vi "Prober_InitialiseUI.vi"(8 "error in (no error)":errorcluster, 11 "ProbeStationControl in":refnum<class "ProbeStationControl.lvclass">) -> (0 "error out":errorcluster, 3 "ProbeStationControl out":refnum<class "ProbeStationControl.lvclass">)   [LabVIEW 2018, in "ProbeStationControl.lvclass"]
uses:
  ProbeStationControl.lvclass
  ProbeStationControl.lvclass/ProbeStationControl.ctl
panel:
  in  "Needles Clear":bool
  in  "Nucleus":bool
  in  "Stop Button":bool
  out "Ref No.":u32
  # "Starting Probe Station Control Interface"
  # "Before continuing, please confirm the following:"
  # "1. NUCLEUS is activiated"
  # "2. No device on chuck and needles are clear"
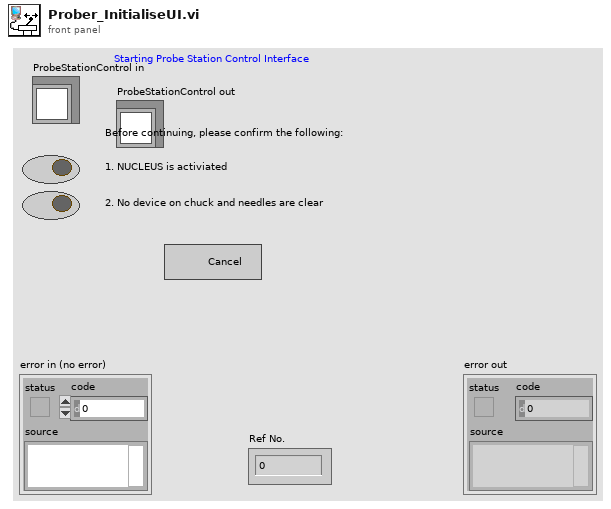
[diagram p1: front panel]
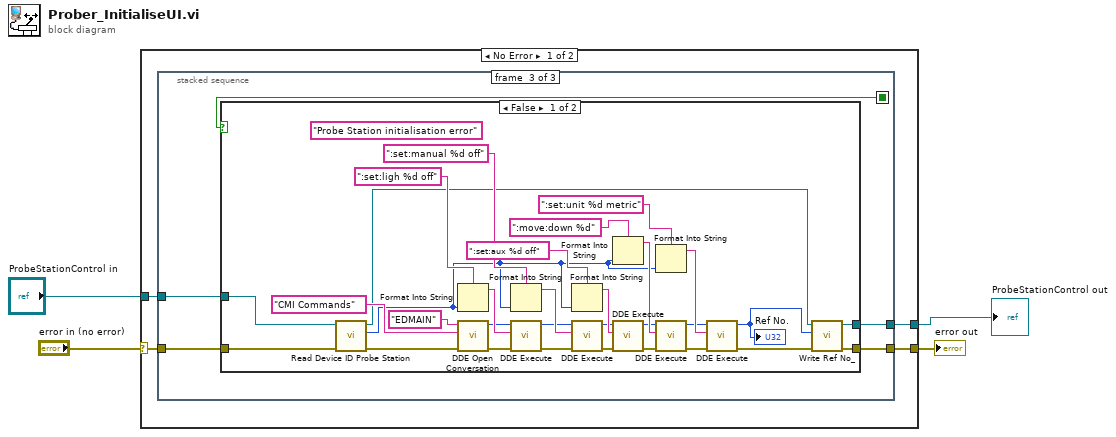
[diagram p0: block diagram]
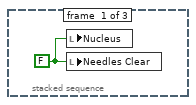
[diagram p2: hidden frame]
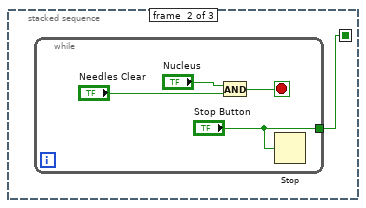
[diagram p3: hidden frame]
diagram:
  n1 = case shown="No Error" "error in (no error)" {
    selector: "error in (no error)" -> [w8 w54]
    tunnel: [w6 w54] -> w3
    tunnel: "ProbeStationControl in" -> [w7 w53]
    tunnel: [w5 w53] -> w1
    frame No Error {
      n2 = stacked-sequence {
        seq-local: [_ w10 _] -> [_ _ w19]
        tunnel: w8 -> [_ _ w17]
        tunnel: w7 -> [_ _ w18]
        tunnel: [_ _ w16] -> w6
        tunnel: [_ _ w15] -> w5
        frame #0 {
          w9 = FALSE
          n3 = local write "Nucleus"(w9) -> ()
          n4 = local write "Needles Clear"(w9) -> ()
        }
        frame #1 {
          n5 = while {
            tunnel: ["Stop Button"] -> w10
            stop <- w12 stop-if-true
            n6 = And(x="Nucleus", y="Needles Clear") -> (x .and. y?=w12:bool)
            n7 = Stop(stop? (T)="Stop Button") -> ()
          }
        }
        frame #2 {
          n8 = case shown="False" w19 {
            tunnel: w18 -> [w28 w51]
            tunnel: w17 -> [w27 w52]
            tunnel: [w22 w52] -> w16
            tunnel: [w20 w51] -> w15
            frame False {
              (unwired) "Probe Station initialisation error" ("Error String IN")
              n9 = call "Read Device ID Probe Station.vi"("error in (no error)"=w27, "ProbeStationControl in"=w28) -> ("error out"=w24:errorcluster, "Device ID Probe Station"=w26:u32, "ProbeStationControl out"=w25:refnum<class "ProbeStationControl.lvclass">)  [unwired: 7 in]
              n10 = Format Into String(format string=":set:ligh %d off", w26) -> (resulting string=w46:string)  [unwired: 2 in, 1 out]
              n11 = call <vilib>:"DDE Open Conversation.vi"("error in (no error)"=w24, "topic"="CMI Commands", "service"="EDMAIN") -> ("error out"=w30:errorcluster, "conversation refnum"=w29:u32)  [unwired: 5 in]
              n12 = Format Into String(format string=":set:manual %d off" ("command"), w26) -> (resulting string=w43:string)  [unwired: 2 in, 1 out]
              n13 = call <vilib>:"DDE Execute.vi"("error in (no error)"=w30, "command"=w46, "conversation refnum in"=w29) -> ("error out"=w34:errorcluster, "conversation refnum out"=w31:u32)  [unwired: 5 in]
              n14 = Format Into String(format string=":set:aux %d off" ("command"), w26) -> (resulting string=w44:string)  [unwired: 2 in, 1 out]
              n15 = call <vilib>:"DDE Execute.vi"("error in (no error)"=w34, "command"=w43, "conversation refnum in"=w31) -> ("error out"=w35:errorcluster, "conversation refnum out"=w32:u32)  [unwired: 5 in]
              n16 = Format Into String(format string=":move:down %d" ("command"), w26) -> (resulting string=w45:string)  [unwired: 2 in, 1 out]
              n17 = call <vilib>:"DDE Execute.vi"("error in (no error)"=w35, "command"=w44, "conversation refnum in"=w32) -> ("error out"=w36:errorcluster, "conversation refnum out"=w33:u32)  [unwired: 5 in]
              n18 = Format Into String(format string=":set:unit %d metric" ("command"), w26) -> (resulting string=w50:string)  [unwired: 2 in, 1 out]
              n19 = call <vilib>:"DDE Execute.vi"("error in (no error)"=w36, "command"=w45, "conversation refnum in"=w33) -> ("error out"=w47:errorcluster, "conversation refnum out"=w48:u32)  [unwired: 5 in]
              n20 = call <vilib>:"DDE Execute.vi"("error in (no error)"=w47, "command"=w50, "conversation refnum in"=w48) -> ("error out"=w23:errorcluster, "conversation refnum out"=w21:u32)  [unwired: 5 in]
              "Ref No." <- w21
              n21 = call "Write Ref No_.vi"("error in (no error)"=w23, "Ref No."=w21, "ProbeStationControl in"=w25) -> ("error out"=w22:errorcluster, "ProbeStationControl out"=w20:refnum<class "ProbeStationControl.lvclass">)  [unwired: 7 in]
            }
            frame True {
            }
          }
        }
      }
    }
    frame Error {
    }
  }
  "error out" <- w3
  "ProbeStationControl out" <- w1
